vi "create report string.vi"(11 "failure":T1 {"code" format="%.0x"}) -> (0 "error out":errorcluster, 3 "report string":string)   [LabVIEW 2013]
uses:
  failure.ctl
  <vilib>/addons/JSON API/Variant JSON/Variant JSON.lvlib
  <vilib>/addons/JSON API/JSON Value/JSON Value.lvclass
  <vilib>/addons/JSON API/JSON Object/JSON Object.lvclass
  <vilib>/addons/JSON API/JSON Scalar/JSON Scalar.lvclass
  failure.lvlib
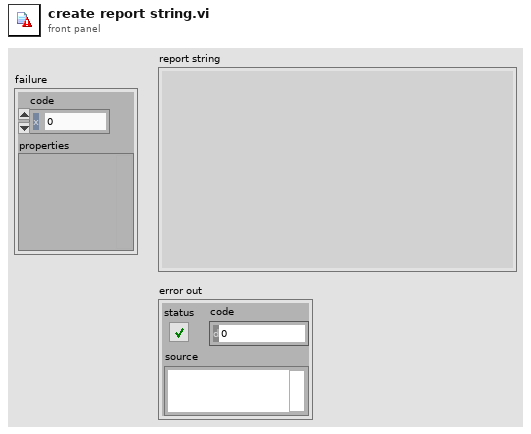
[diagram p1: front panel]
types:
  T1 = typedef "failure.lvlib/failure.ctl" = cluster{"code":i32, "properties":variant}
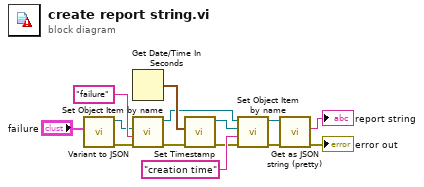
[diagram p0: block diagram]
diagram:
  n1 = call <vilib>:"Variant to JSON.vi"("Variant"="failure") -> ("error out"=w5:errorcluster, "JSON Value out"=w4:refnum<class "JSON Value.lvclass">)  [unwired: 9 in]
  n2 = Get Date/Time In Seconds() -> (seconds since 1Jan1904=w12:timestamp)
  n3 = call <vilib>:"Set Object Item by name.vi"("error in (no error)"=w5, "name"="failure", "Value"=w4) -> ("error out"=w8:errorcluster, "JSON Object out"=w7:refnum<class "JSON Object.lvclass">)  [unwired: 6 in, 1 out]
  n4 = call <vilib>:"Set Timestamp.vi"("error in (no error)"=w8, "Time Stamp"=w12) -> ("error out"=w9:errorcluster, "JSON Scalar out"=w10:refnum<class "JSON Scalar.lvclass">)  [unwired: 8 in]
  n5 = call <vilib>:"Set Object Item by name.vi"("error in (no error)"=w9, "name"="creation time", "Value"=w10, "JSON Object in"=w7) -> ("error out"=w13:errorcluster, "JSON Object out"=w14:refnum<class "JSON Object.lvclass">)  [unwired: 5 in, 1 out]
  n6 = call <vilib>:"Get as JSON string (pretty).vi"("error in (no error)"=w13, "JSON Value in"=w14) -> ("error out"=→"error out":errorcluster, "String"=→"report string":string)  [unwired: 8 in]
